vi "PulseGenRetrig.vi"(2 "idle state":i32(ring)=10214 items=["High"=10192, "Low"=10214], 3 "source":tag, 4 "error in":errorcluster, 5 "high time":dbl, 6 "pulse delay (s or cycles)":dbl, 7 "counter":tag) -> (0 "error out":errorcluster, 1 "task out":refnum<k21>)   [LabVIEW 2022 SP3]
uses:
  <vilib>/DAQmx/create/channels.llb/DAQmx Create Channel (CO-Pulse Generation-Time).vi
  <vilib>/DAQmx/configure/trigger.llb/DAQmx Start Trigger (Digital Edge).vi
  <resource>/objmgr/daqmx.rc
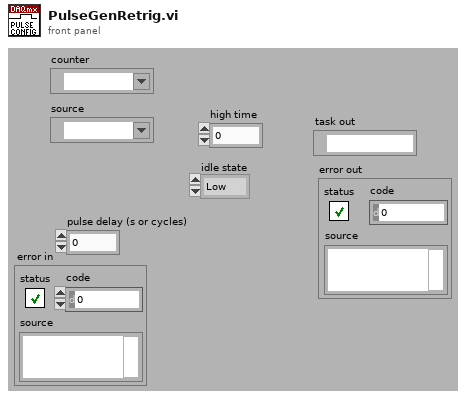
[diagram p1: front panel]
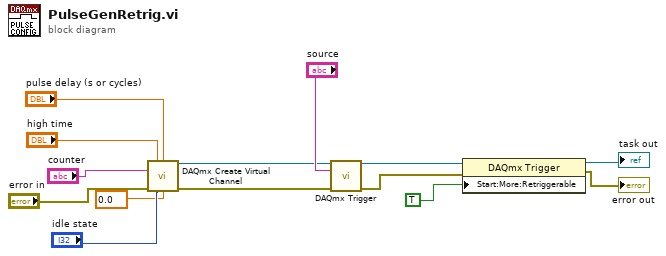
[diagram p0: block diagram]
diagram:
  n1 = call-poly <vilib>:"DAQmx Create Virtual Channel.vi"("high time"="high time", "low time"="pulse delay (s or cycles)", "counter"="counter", "error in"="error in", "idle state"="idle state", "initial delay"=0.0) -> ("task out"=w1:refnum<k21>, "error out"=w3:errorcluster)  [unwired: 3 in, 5 out]
  n2 = call-poly <vilib>:"DAQmx Trigger.vi"("task/channels in"=w1, "source"="source", "error in"=w3) -> ("task out"=w11:refnum<k21>, "error out"=w12:errorcluster)  [unwired: 1 in, 10 out]
  n3 = property class="DAQmx Trigger"(reference=w11, error in=w12, "Start:More:Retriggerable"=TRUE) -> (reference out=→"task out":refnum<k21>, error out=→"error out":errorcluster)
